vi "stp.vi"(11 "Speed":dbl[](array[numeric])) -> (0 "Out 4":dbl format="%#_13g", 1 "Out 3":dbl format="%#_13g", 2 "Out 2":dbl format="%#_13g", 3 "Out 1":dbl format="%#_13g")   [LabVIEW 2015]
uses:
  <vilib>/imath/engines/lvmath2/RunTimeEngine/ArithmeticOperatorToken/NIMS_ArithmeticOperator_power(S).vi
  <instcachedir>/0/NIMS_ArithmeticOperator_power(S)_DFB67823F1414E5097C86E39787D8CA8.lvgen/NIMS_ArithmeticOperator_power(S)_DFB67823F1414E5097C86E39787D8CA8_014.vi
  <vilib>/imathl/engines/lvmath/Functions/Error Handling/Create Error.vi
  <vilib>/imath/engines/lvmath2/RunTimeEngine/NodeEndStatement/NIMS_NodeEndStatement_Output.vi
  <instcachedir>/0/NIMS_NodeEndStatement_Output_53EC0D466D134D7ABD903AC30B43404B.lvgen/NIMS_NodeEndStatement_Output_53EC0D466D134D7ABD903AC30B43404B_009.vi
  <vilib>/imath/engines/lvmath2/RunTimeEngine/ErrorHandling/NIMS_Finalize Error.vi
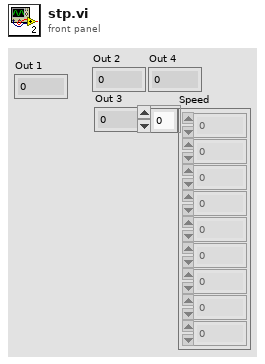
[diagram p1: front panel]
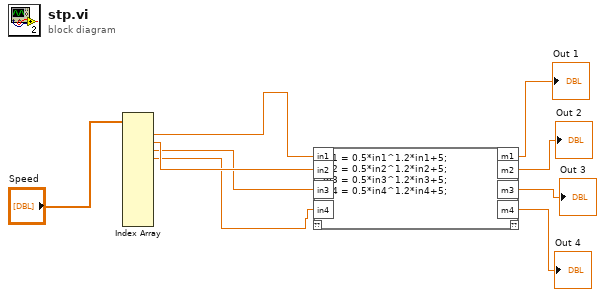
[diagram p0: block diagram]
diagram:
  n1 = Index Array ("Index Array 7")(array="Speed") -> (element #1=w5:dbl, element #2=w3:dbl, element #3=w2:dbl, element #4=w1:dbl)  [unwired: 12 in, 8 out]
  n2 = mathscript code="m1 = 0.5*in1^1.2*in1+5;\nm2 = 0.5*in2^1.2*in2+5;\nm3 = 0.5*in3^1.2*in3+5;\nm4 = 0.5*in4^1.2*in4+5;"("in1"=w5, "in2"=w3, "in3"=w2, "in4"=w1) -> ("m1"=→"Out 1":cdb, "m2"=→"Out 2":cdb, "m3"=→"Out 3":cdb, "m4"=→"Out 4":cdb)  [unwired: 1 in, 1 out]
